vi "Timestamp_HMS.vi"() -> (0 "Current Time":string)   [LabVIEW 2024]
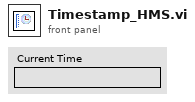
[diagram p1: front panel]
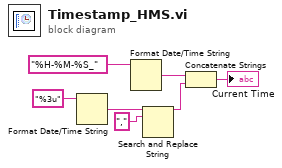
[diagram p0: block diagram]
diagram:
  n1 = Format Date/Time String(time format string (%c)="%3u") -> (date/time string=w2:string)  [unwired: 2 in]
  n2 = Format Date/Time String(time format string (%c)="%H-%M-%S_") -> (date/time string=w3:string)  [unwired: 2 in]
  n3 = Search and Replace String(input string=w2, search string=",") -> (result string=w1:string)  [unwired: 6 in, 3 out]
  n4 = Concatenate Strings(w3, w1) -> (→"Current Time":string)
